vi "Write Class Name.vi"(5 "Class Name":string, 9 "Generic in":refnum<class "Generic.lvclass">) -> (3 "Generic out":refnum<class "Generic.lvclass">)   [LabVIEW 2014, in "Raspberry Pi Compatible Compiler for LabVIEW.lvlib" / "Generic.lvclass"]
uses:
  Generic.lvclass
  Generic.lvclass/Generic.ctl
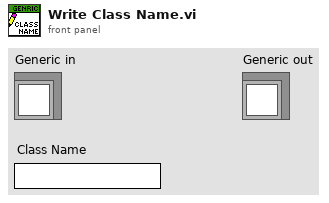
[diagram p1: front panel]
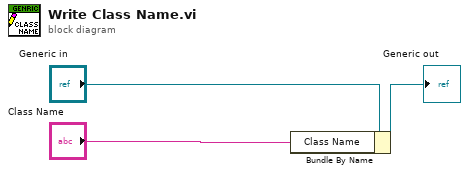
[diagram p0: block diagram]
diagram:
  n1 = Bundle By Name(cluster="Generic in", "Class Name"="Class Name") -> (→"Generic out":refnum<class "Generic.lvclass">)
